vi "2D Cross Correlation (CDB).vi"(9 "algorithm":enum32{"direct", "frequency domain"}(ring)=enum."frequency domain", 10 "Y":cdb[][](array[numeric]), 11 "X":cdb[][](array[numeric])) -> (0 "error":i32, 3 "Rxy":cdb[][](array[numeric]))   [LabVIEW 2017, in "NI_AALPro.lvlib"]
doc: "Computes the cross correlation of the input sequences <B>X</B> and <B>Y</B>. Wire data to the <B>X</B> and <B>Y</B> inputs to determine the polymorphic instance to use or manually select the instance."
uses:
  NI_AALPro.lvlib
  lvanlys.dll
panel:
  # "2D CrossCorrelation (CDB)"
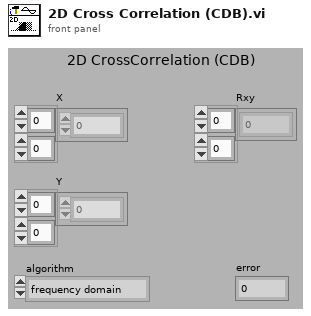
[diagram p1: front panel]
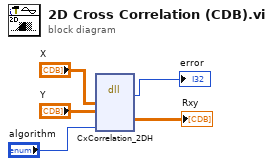
[diagram p0: block diagram]
diagram:
  n1 = dll-call lib="C:/Program Files/National Instruments/LabVIEW 2017/resource/lvanlys.*" fn="CxCorrelation_2DH"("X"="X", "Y"="Y", "domain"="algorithm") -> (→"error":i32, "Rxy"=→"Rxy":cdb[][])  [unwired: 7 in, 2 out]
